vi "Day04-02_중복 데이터, 데이터 손실.vi"() -> ()   [LabVIEW 2021]
panel:
  in  "불리언":bool
  out "데이터 손실":dbl(graph)
  out "중복 데이터":dbl(graph)
  out "반복 터미널 값 2":dbl
  out "반복 터미널 값":dbl
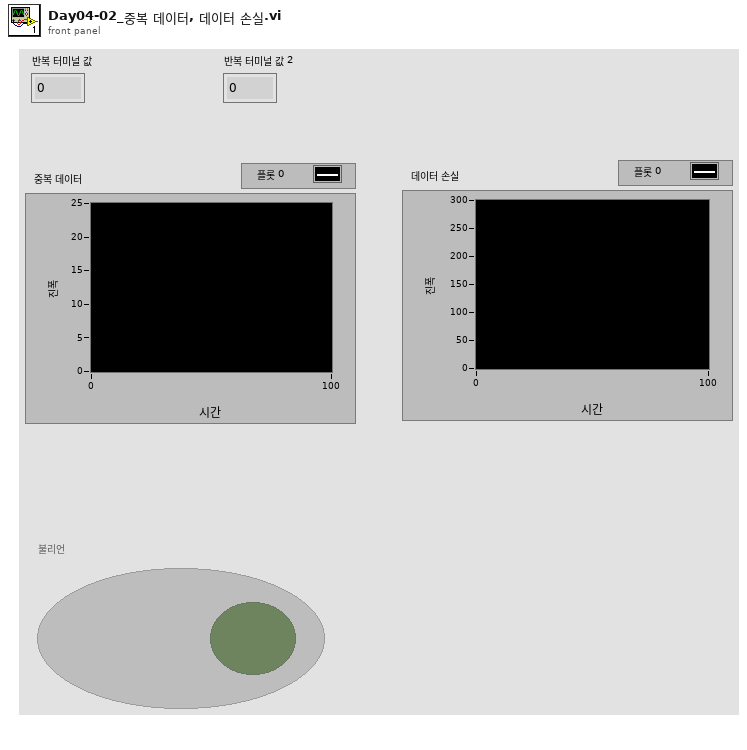
[diagram p1: front panel]
types:
  T1 = enum8{"Enabled", "Disabled", "Disabled and Grayed Out"}
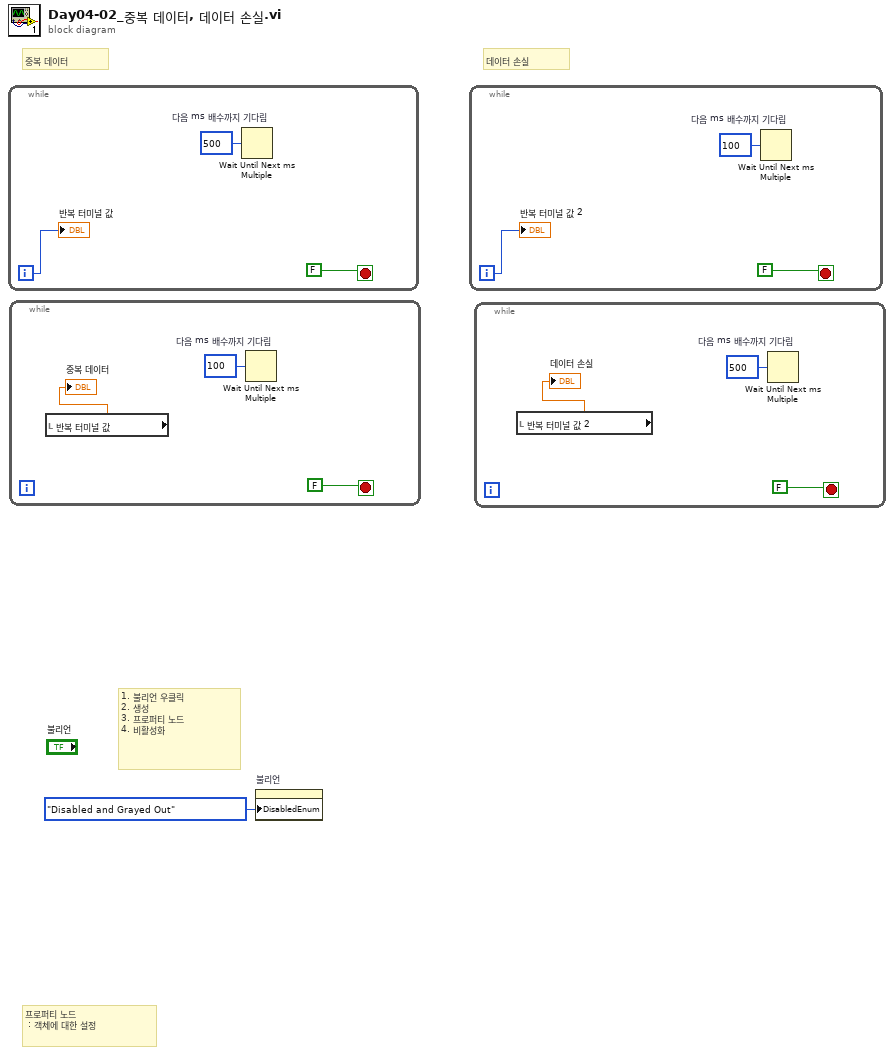
[diagram p0: block diagram]
diagram:
  # "프로퍼티 노드\n : 객체에 대한 설정"
  # "1. 불리언 우클릭 \n2. 생성\n3. 프로퍼티 노드\n4. 비활성화"
  # "데이터 손실"
  # "중복 데이터"
  n1 = while {
    i -> [w4]
    stop <- FALSE stop-if-true
    n2 = Wait Until Next ms Multiple "다음 ms 배수까지 기다림"(millisecond multiple=u32 500 ("ms 배수")) -> ()  [unwired: 1 out]
    "반복 터미널 값" <- w4
  }
  n3 = while {
    stop <- FALSE stop-if-true
    n4 = local read "반복 터미널 값"() -> (→"중복 데이터":dbl)
    n5 = Wait Until Next ms Multiple "다음 ms 배수까지 기다림"(millisecond multiple=u32 100 ("ms 배수")) -> ()  [unwired: 1 out]
  }
  n6 = property on="불리언" class="Bool (엄격한)"("DisabledEnum"=T1."Disabled and Grayed Out" ("비활성화")) -> ()  [unwired: 2 in, 2 out]
  n7 = while {
    i -> [w10]
    stop <- FALSE stop-if-true
    n8 = Wait Until Next ms Multiple "다음 ms 배수까지 기다림"(millisecond multiple=u32 100 ("ms 배수")) -> ()  [unwired: 1 out]
    "반복 터미널 값 2" <- w10
  }
  n9 = while {
    stop <- FALSE stop-if-true
    n10 = local read "반복 터미널 값 2"() -> (→"데이터 손실":dbl)
    n11 = Wait Until Next ms Multiple "다음 ms 배수까지 기다림"(millisecond multiple=u32 500 ("ms 배수")) -> ()  [unwired: 1 out]
  }
